vi "UI Create.vi"(8 "error in (no error)":errorcluster, 10 "VI Refnum":refnum<vi>, 11 "Button_UI in":refnum<class "Button_UI.lvclass">) -> (0 "error out":errorcluster, 3 "Button_UI out":refnum<class "Button_UI.lvclass">)   [LabVIEW 2015, in "Button_UI.lvclass"]
uses:
  Button_UI.lvclass
  GUI Control/Type Definition/UI Maker State Variable.ctl
  <vilib>/Utility/miscctls.llb/LVPointTypeDef.ctl
  GUI Control/GUI Control.lvclass/GUI Control.ctl
  Button_UI.lvclass/Button_UI.ctl
  GUI Control/GUI Control.lvclass
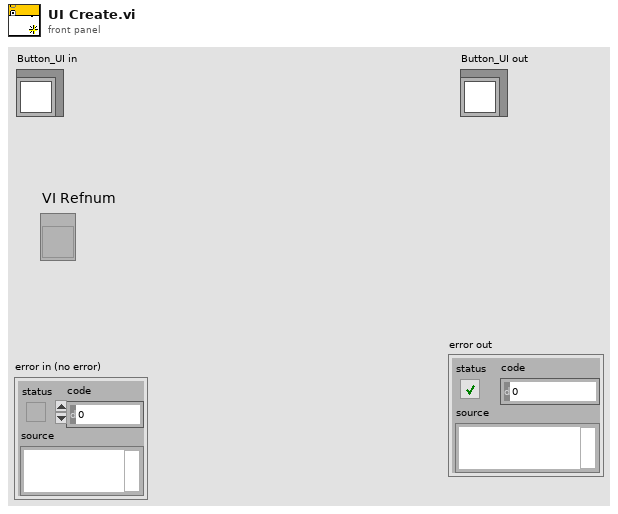
[diagram p1: front panel]
types:
  T1 = typedef "UI Maker State Variable.ctl" = enum16{"Start Undo", "Generate Control", "Configure Control ", "Configure Control Part", "End Undo"}
  T2 = typedef "LVPointTypeDef.ctl" = cluster{"Horizontal":i16, "Vertical":i16}
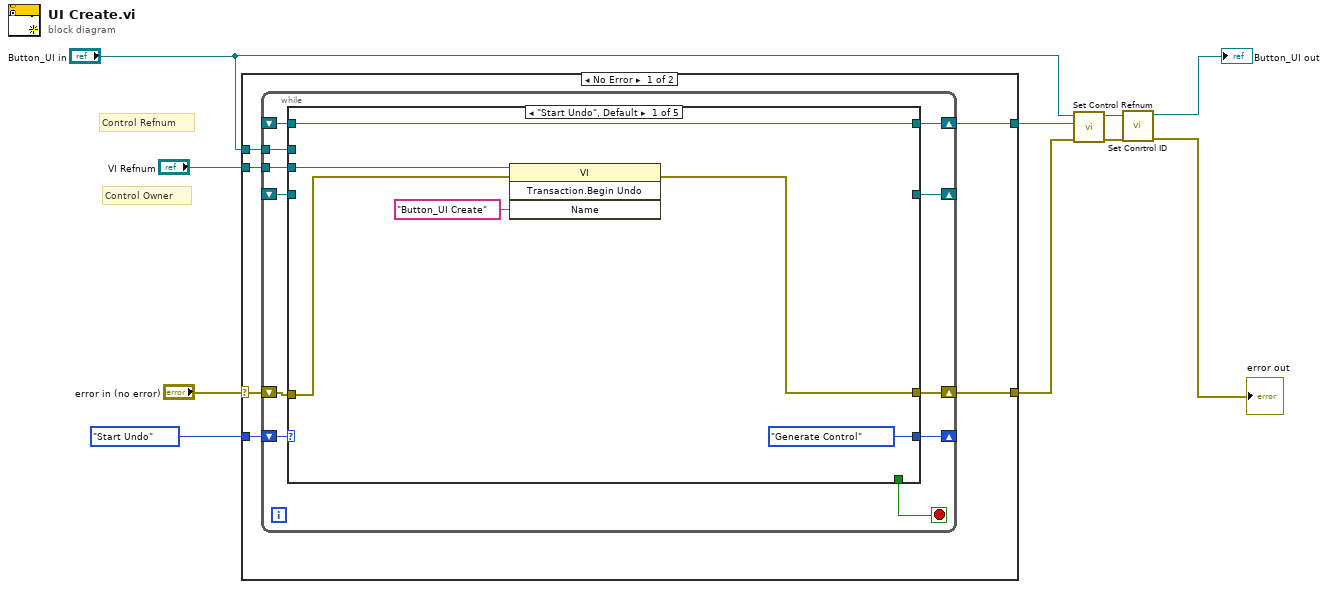
[diagram p0: block diagram]
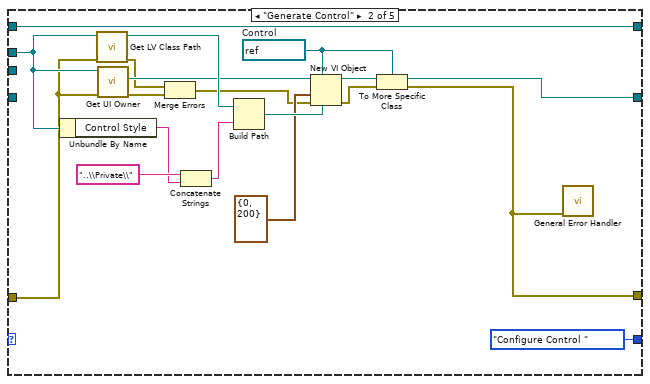
[diagram p2: hidden frame]
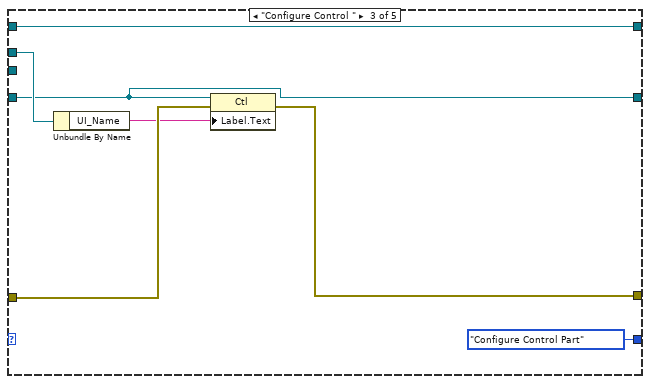
[diagram p3: hidden frame]
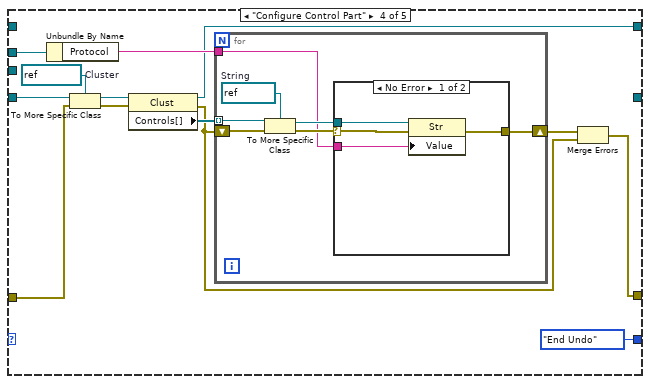
[diagram p4: hidden frame]
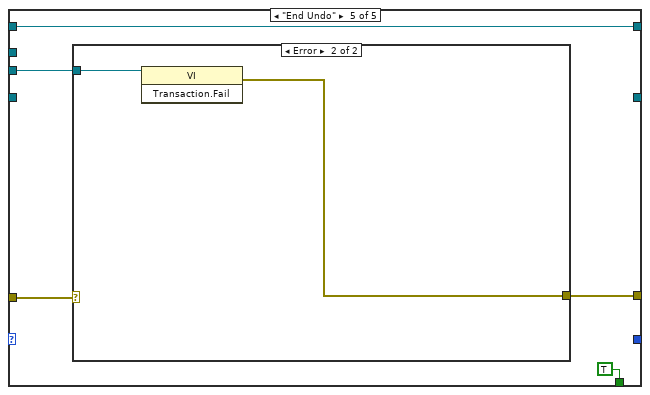
[diagram p6: hidden frame]
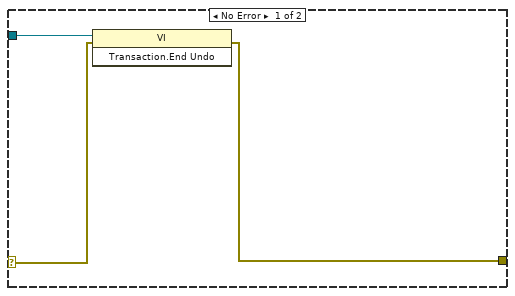
[diagram p7: hidden frame]
diagram:
  # "Control Refnum"
  # "Control Owner"
  n1 = case shown="No Error" "error in (no error)" {
    selector: "error in (no error)" -> [w12 w94]
    tunnel: UI_Maker_State_Variable."Start Undo" -> [w16 _]
    tunnel: "VI Refnum" -> [w15 _]
    tunnel: "Button_UI in" -> [w14 _]
    tunnel: [w13 w94] -> w5
    tunnel: [w11 _] -> w6
    frame No Error {
      n2 = while {
        tunnel: w15 -> [w26]
        tunnel: w14 -> [w23]
        shift-right: [w22] -> _
        shift-left: w16 -> [w27]
        shift-right: [w24] -> w13
        shift-left: w12 -> [w25]
        shift-right: [w21] -> _
        shift-left: _ -> [w20]
        shift-right: [w18] -> w11
        shift-left: _ -> [w17]
        stop <- w19 stop-if-true
        n3 = case shown="\"Start Undo\", Default" w27 {
          tunnel: w26 -> [w33 _ _ _ w87]
          tunnel: w25 -> [w32 w38 w58 w70 w88]
          tunnel: [w30 w41 w56 w62 w86] -> w24
          tunnel: w23 -> [_ w40 w59 w66 _]
          tunnel: [UI_Maker_State_Variable."Generate Control" UI_Maker_State_Variable."Configure Control " UI_Maker_State_Variable."Configure Control Part" UI_Maker_State_Variable."End Undo" _] -> w22
          tunnel: [_ w43 w55 _ _] -> w21
          tunnel: w20 -> [_ _ w55 w72 _]
          tunnel: [_ _ _ _ TRUE] -> w19
          tunnel: [w28 w34 w53 w60 w84] -> w18
          tunnel: w17 -> [w28 w34 w53 _ w84]
          frame "Start Undo", Default {
            n4 = invoke class="VI" method="Transaction.Begin Undo"(reference=w33, error in=w32, "Name"="Button_UI Create") -> (error out=w30:errorcluster)  [unwired: 1 in, 3 out]
          }
          frame "Generate Control" {
            w46 = refnum<vi> refnum  # Control
            n5 = Unbundle By Name(w40) -> ("Control Style"=w50:string)
            n6 = call <vilib>:"Get LV Class Path.vi"("error in (no error)"=w38, "object"=w40) -> ("error out"=w37:errorcluster, "class path"=w52:path)  [unwired: 8 in]
            n7 = call "Get UI Owner.vi"("error in (no error)"=w38, "GUI Control in"=w40) -> ("error out"=w36:errorcluster, "Owner"=w39:refnum<vi>)  [unwired: 7 in, 1 out]
            n8 = Merge Errors(w37, w36) -> (w35:errorcluster)
            n9 = Concatenate Strings("..\\Private\\" ("string"), w50) -> (w49:string)
            n10 = Build Path(base path=w52, name or relative path=w49) -> (appended path=w48:path)
            n11 = New VI Object(vi object class=w46, owner refnum=w39, position/next to=T2 {"Horizontal"=0, "Vertical"=200} ("location"), 6:w48, 8:w35) -> (object refnum=w47:refnum<vi>, 0:w45:errorcluster)  [unwired: 3 in]
            n12 = To More Specific Class(target class=w46, reference=w47, error in=w45) -> (specific class reference=w43:refnum<vi>, error out=w41:errorcluster)
            n13 = call <vilib>:"General Error Handler.vi"("error in (no error)"=w41) -> ()  [unwired: 10 in, 5 out]
          }
          frame "Configure Control " {
            n14 = Unbundle By Name(w59) -> ("UI_Name"=w57:string)
            n15 = property class="Ctl"(reference=w55, error in=w58, "Label.Text"=w57) -> (error out=w56:errorcluster)  [unwired: 1 out]
          }
          frame "Configure Control Part" {
            w71 = refnum<vi> refnum  # Cluster
            n16 = Unbundle By Name(w66) -> ("Protocol"=w65:string)
            n17 = To More Specific Class(target class=w71, reference=w72, error in=w70) -> (specific class reference=w69:refnum<vi>, error out=w68:errorcluster)
            n18 = property class="Clust"(reference=w69, error in=w68) -> (reference out=w60:refnum<vi>, error out=w63:errorcluster, "Controls[]"=w67:refnum<vi>[])
            n19 = for {
              tunnel: w67 -> [w79] mode=indexing
              tunnel: w65 -> [w74]
              shift-right: [w73] -> w64
              shift-left: w63 -> [w78]
              w77 = refnum<vi> refnum  # String
              n20 = To More Specific Class(target class=w77, reference=w79, error in=w78) -> (specific class reference=w75:refnum<vi>, error out=w76:errorcluster)
              n21 = case shown="No Error" w76 {
                selector: w76 -> [w82 _]
                tunnel: w75 -> [w83 _]
                tunnel: w74 -> [w81 _]
                tunnel: [w80 _] -> w73
                frame No Error {
                  n22 = property class="Str"(reference=w83, error in=w82, "Value"=w81) -> (error out=w80:errorcluster)  [unwired: 1 out]
                }
                frame Error {
                }
              }
            }
            n23 = Merge Errors(w64, w63) -> (w62:errorcluster)
          }
          frame "End Undo" {
            n24 = case shown="Error" w88 {
              selector: w88 -> [w90 _]
              tunnel: w87 -> [w91 w93]
              tunnel: [w89 w92] -> w86
              frame No Error {
                n25 = invoke class="VI" method="Transaction.End Undo"(reference=w91, error in=w90) -> (error out=w89:errorcluster)  [unwired: 1 in, 2 out]
              }
              frame Error {
                n26 = invoke class="VI" method="Transaction.Fail"(reference=w93) -> (error out=w92:errorcluster)  [unwired: 2 in, 2 out]
              }
            }
          }
        }
      }
    }
    frame Error {
    }
  }
  n27 = call "Set Control Refnum.vi"("error in (no error)"=w5, "Ctl Refnum"=w6, "GUI Control in"="Button_UI in") -> ("error out"=w3:errorcluster, "GUI Control out"=w4:refnum<class "Button_UI.lvclass">)  [unwired: 7 in]
  n28 = call "Set Conrtrol ID.vi"("error in (no error)"=w3, "GUI Control in"=w4) -> ("error out"=→"error out":errorcluster, "GUI Control out"=→"Button_UI out":refnum<class "Button_UI.lvclass">)  [unwired: 8 in]
